vi "serialization tests.vi"() -> ()   [LabVIEW 2013, in "Scaling tests.lvlib"]
uses:
  Scaling tests.lvlib
  module/configuration/Scaling configuration.lvclass
panel:
  out "modules equal":bool
  out "channels equal":bool
  out "no error":errorcluster
  out "no error":errorcluster
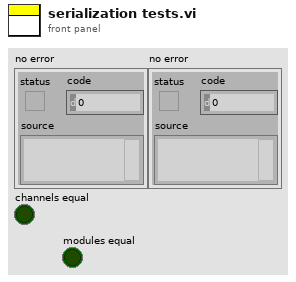
[diagram p1: front panel]
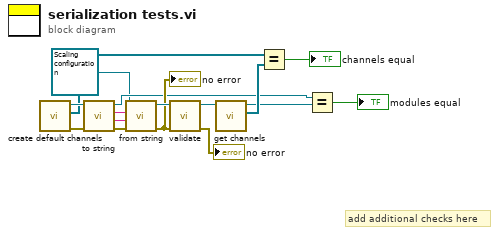
[diagram p0: block diagram]
diagram:
  # "add additional checks here"
  n1 = call "create default channels.vi"() -> ("error out"=w6:errorcluster, "channels"=w5:refnum<class "TBM channel.lvclass">[], "module"=w7:refnum<class "Scaling configuration.lvclass">)  [unwired: 7 in, 2 out]
  n2 = call-dynamic "to string.vi"("error in"=w6, "Scaling configuration in"=w7) -> ("error out"=w16:errorcluster, "data"=w15:string, "version"=w14:string, "Scaling configuration out"=w2:refnum<class "Scaling configuration.lvclass">)  [unwired: 6 in]
  n3 = call-dynamic "from string.vi"("error in"=w16, "data"=w15, "version"=w14, "Scaling configuration in"=refnum<class "Scaling configuration.lvclass"> refnum ("tag bus configurable plugin module configuration")) -> ("error out"=w11:errorcluster, "Scaling configuration out"=w13:refnum<class "Scaling configuration.lvclass">)  [unwired: 6 in]
  "no error" <- w11
  n4 = call-dynamic "validate.vi"("error in"=w11, "Scaling configuration in"=w13) -> ("error out"=→"no error":errorcluster, "Scaling configuration out"=w9:refnum<class "Scaling configuration.lvclass">)  [unwired: 8 in]
  n5 = call-dynamic "get channels.vi"("Scaling configuration in"=w9) -> ("channels"=w8:refnum<class "TBM channel.lvclass">[], "Scaling configuration out"=w3:refnum<class "Scaling configuration.lvclass">)  [unwired: 9 in]
  n6 = Equal?(x=w5, y=w8) -> (x = y?=→"channels equal":bool)
  n7 = Equal?(x=w2, y=w3) -> (x = y?=→"modules equal":bool)
